vi "Graphics-Draw Wedge.vi"(0 "Picture In":picture, 5 "Angle (cycles)":dbl, 7 "Width (cycles)":dbl=0.025, 9 "Radius (pixels)":dbl=205.0, 11 "Thickness (fraction)":dbl=0.2, 12 "Fill color":u32(colorbox)=16860, 13 "Line color":u32(colorbox), 14 "Line width":i32=1) -> (4 "Picture Out":picture)   [LabVIEW 2015]
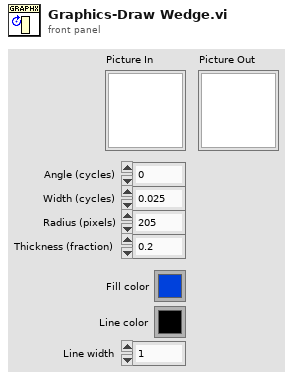
[diagram p1: front panel]
types:
  T1 = enum32{"Solid", "Dash", "Dot", "DashDot", "DashDotDot"}
  T2 = cluster{"Line width":i32, "Style":enum32{"Solid", "Dash", "Dot", "DashDot", "DashDotDot"}}
  T3 = cluster{"Radius (pixels)":dbl, "Radius (pixels)":dbl}
  T4 = cluster{"Radius (pixels)":i16, "Radius (pixels)":i16}
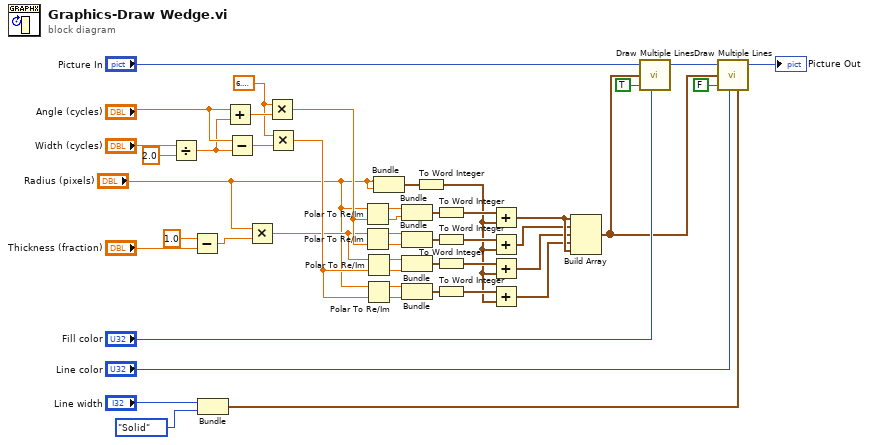
[diagram p0: block diagram]
diagram:
  w41 = 6.283185307179586
  n1 = Divide(x="Width (cycles)", y=2.0) -> (x/y=w44:dbl)
  n2 = Subtract(x=1.0, y="Thickness (fraction)") -> (x-y=w39:dbl)
  n3 = Bundle("Line width"="Line width", "Style"=T1."Solid") -> (w11:T2)  [unwired: 1 in]
  n4 = Add(x="Angle (cycles)", y=w44) -> (x+y=w43:dbl)
  n5 = Subtract(x="Angle (cycles)", y=w44) -> (x-y=w42:dbl)
  n6 = Multiply(x="Radius (pixels)", y=w39) -> (x*y=w23:dbl)
  n7 = Multiply(x=w41, y=w43) -> (x*y=w37:dbl)
  n8 = Multiply(x=w41, y=w42) -> (x*y=w36:dbl)
  n9 = Polar To Re/Im(2:w37, 3:"Radius (pixels)") -> (0:w34:dbl, 1:w35:dbl)
  n10 = Polar To Re/Im(2:w37, 3:w23) -> (0:w30:dbl, 1:w31:dbl)
  n11 = Polar To Re/Im(2:w36, 3:w23) -> (0:w26:dbl, 1:w27:dbl)
  n12 = Polar To Re/Im(2:w36, 3:"Radius (pixels)") -> (0:w24:dbl, 1:w25:dbl)
  n13 = Bundle("Radius (pixels)"="Radius (pixels)", "Radius (pixels)"="Radius (pixels)") -> (w9:T3)  [unwired: 1 in]
  n14 = Bundle(w35, w34) -> (w33:cluster{dbl, dbl})  [unwired: 1 in]
  n15 = Bundle(w31, w30) -> (w32:cluster{dbl, dbl})  [unwired: 1 in]
  n16 = Bundle(w27, w26) -> (w29:cluster{dbl, dbl})  [unwired: 1 in]
  n17 = Bundle(w25, w24) -> (w28:cluster{dbl, dbl})  [unwired: 1 in]
  n18 = To Word Integer(number=w9) -> (16bit integer=w4:T4)
  n19 = To Word Integer(number=w33) -> (16bit integer=w22:cluster{i16, i16})
  n20 = To Word Integer(number=w32) -> (16bit integer=w7:cluster{i16, i16})
  n21 = To Word Integer(number=w29) -> (16bit integer=w6:cluster{i16, i16})
  n22 = To Word Integer(number=w28) -> (16bit integer=w5:cluster{i16, i16})
  n23 = Add(x=w22, y=w4) -> (x+y=w8:cluster{i16, i16})
  n24 = Add(x=w7, y=w4) -> (x+y=w3:cluster{i16, i16})
  n25 = Add(x=w6, y=w4) -> (x+y=w2:cluster{i16, i16})
  n26 = Add(x=w5, y=w4) -> (x+y=w1:cluster{i16, i16})
  n27 = Build Array(w8, w3, w2, w1, w8) -> (w15:cluster{i16, i16}[])
  n28 = call <vilib>:"Draw Multiple Lines.vi"("picture"="Picture In", "line endpoints"=w15, "fill?(F)"=TRUE, "color(black)"="Fill color") -> ("new picture"=w18:picture)  [unwired: 5 in]
  n29 = call <vilib>:"Draw Multiple Lines.vi"("picture"=w18, "line endpoints"=w15, "fill?(F)"=FALSE, "color(black)"="Line color", "pen"=w11) -> ("new picture"=→"Picture Out":picture)  [unwired: 4 in]
